vi "RT Controller.vi"() -> ()   [LabVIEW 2017]
uses:
  <vilib>/LabVIEW Targets/FPGA/cRIO/shared/nicrio_ModuleControls/nicrio_cRIO-9775_RecordDataRates4ChansRing.ctl
  <vilib>/FPGAPlugInAG/cRIO-9063/niLvFpga_Open_cRIO-9063.vi
  <vilib>/rvi/interface/common/dynamic/niFpgaDynamicAddResources.vi
  <vilib>/FPGAPlugInAG/Dynamic/niLvFpga_Reset_Dynamic.vi
  <vilib>/Utility/error.llb/Error Cluster From Error Code.vi
  <vilib>/rvi/errors/niLvFpgaAdjustHostInterfaceError.vi
  <vilib>/FPGAPlugInAG/Dynamic/niLvFpga_Run_Dynamic.vi
  <vilib>/RVI Host/nirviSupport.llb/nirviErrorClusterFromErrorCode.vi
  <vilib>/FPGAPlugInAG/Dynamic/niLvFpga_Close_Dynamic.vi
  <vilib>/rvi/interface/nirviOpenFPGA/nirviOpenFPGA.xnode
  FPGA Bitfiles/Mainproject_FPGATarget_Icreadoutclocked_gpGzf-zKHUg.lvbitx
  Ic readout_clocked_dist.vi
  <vilib>/rvi/interface/nirviMethod/nirviMethod.xnode
  <vilib>/rvi/interface/nirviReadWriteControl/nirviReadWriteControl.xnode
  <vilib>/rvi/interface/nirviCloseFPGA/nirviCloseFPGA.xnode
  <resource>/objmgr/ni.dex.rc
  <vilib>/rvi/interface/nirviMethod/StockFPGA_InlinedMethodWaitForSingleIRQ.vi
  <vilib>/FPGAPlugInAG/Dynamic/niLvFpga_WaitOnIrq_Dynamic.vi
  <vilib>/FPGAPlugInAG/Dynamic/niLvFpga_AcknowledgeIrq_Dynamic.vi
  <vilib>/FPGAPlugInAG/Dynamic/niLvFpga_ReadFifo_Dynamic.vi
  <vilib>/rvi/errors/niLvFpgaMergeErrorWithErrorCode.vi
  NiFpgaLv.dll
  <vilib>/rvi/interface/Simulation/niFpgaSimulationCallBeginRW.vi
panel:
  in  "Count ms":u32=15
  out "error out":errorcluster
  in  "Parameters":T2 {"Record Data Rate" items=["20.000 MS/s (NI 9775)"=1, "10.00 MS/s (NI 9775)"=2, "6.667 MS/s (NI 9775)"=3, "5.000 MS/s (NI 9775)"=4, "2.500 MS/s (NI 9775)"=8, "1.667 MS/s (NI 9775)"=12, "1.250 MS/s (NI 9775)"=16, "1.000 MS/s (NI 9775)"=20, "833.333 KS/s (NI 9775)"=24, "714.286 KS/s (NI 9775)"=28, "625.000 KS/s (NI 9775)"=32, "555.556 KS/s (NI 9775)"=36, "500.000 KS/s (NI 9775)"=40, "454.545 KS/s (NI 9775)"=44, "416.667 KS/s (NI 9775)"=48, "384.615 KS/s (NI 9775)"=52, "357.143 KS/s (NI 9775)"=56, "333.333 KS/s (NI 9775)"=60, "312.500 KS/s (NI 9775)"=64, "294.118 KS/s (NI 9775)"=68, "277.778 KS/s (NI 9775)"=72, "263.158 KS/s (NI 9775)"=76, "250.000 KS/s (NI 9775)"=80, "238.095 KS/s (NI 9775)"=84, "227.273 KS/s (NI 9775)"=88, "217.391 KS/s (NI 9775)"=92, "208.333 KS/s (NI 9775)"=96, "200.000 KS/s (NI 9775)"=100, "192.308 KS/s (NI 9775)"=104, "185.185 KS/s (NI 9775)"=108, "178.571 KS/s (NI 9775)"=112, "172.414 KS/s (NI 9775)"=116, "166.667 KS/s (NI 9775)"=120, "161.290 KS/s (NI 9775)"=124, "156.250 KS/s (NI 9775)"=128, "151.515 KS/s (NI 9775)"=132, "147.059 KS/s (NI 9775)"=136, "142.857 KS/s (NI 9775)"=140, "138.889 KS/s (NI 9775)"=144, "135.135 KS/s (NI 9775)"=148, "131.579 KS/s (NI 9775)"=152, "128.205 KS/s (NI 9775)"=156, "125.000 KS/s (NI 9775)"=160, "121.951 KS/s (NI 9775)"=164, "119.048 KS/s (NI 9775)"=168, "116.279 KS/s (NI 9775)"=172, "113.636 KS/s (NI 9775)"=176, "111.111 KS/s (NI 9775)"=180, "108.696 KS/s (NI 9775)"=184, "106.383 KS/s (NI 9775)"=188, "104.167 KS/s (NI 9775)"=192, "102.041 KS/s (NI 9775)"=196, "100.000 KS/s (NI 9775)"=200, "50.000 KS/s (NI 9775)"=400, "33.333 KS/s (NI 9775)"=600, "25.000 KS/s (NI 9775)"=800, "20.000 KS/s (NI 9775)"=1000, "16.667 KS/s (NI 9775)"=1200, "14.286 KS/s (NI 9775)"=1400, "12.500 KS/s (NI 9775)"=1600, "11.111 KS/s (NI 9775)"=1800, "10.000 KS/s (NI 9775)"=2000, "9.091 KS/s (NI 9775)"=2200, "8.333 KS/s (NI 9775)"=2400, "7.692 KS/s (NI 9775)"=2600, "7.143 KS/s (NI 9775)"=2800, "6.667 KS/s (NI 9775)"=3000, "6.250 KS/s (NI 9775)"=3200, "5.882 KS/s (NI 9775)"=3400, "5.556 KS/s (NI 9775)"=3600, "5.000 KS/s (NI 9775)"=4000, "4.762 KS/s (NI 9775)"=4200, "4.545 KS/s (NI 9775)"=4400, "4.348 KS/s (NI 9775)"=4600, "4.167 KS/s (NI 9775)"=4800, "4.000 KS/s (NI 9775)"=5000, "3.846 KS/s (NI 9775)"=5200, "3.571 KS/s (NI 9775)"=5600, "3.333 KS/s (NI 9775)"=6000, "3.125 KS/s (NI 9775)"=6400, "2.941 KS/s (NI 9775)"=6800, "2.778 KS/s (NI 9775)"=7200, "2.632 KS/s (NI 9775)"=7600, "2.500 KS/s (NI 9775)"=8000, "2.381 KS/s (NI 9775)"=8400, "2.273 KS/s (NI 9775)"=8800, "2.174 KS/s (NI 9775)"=9200, "2.083 KS/s (NI 9775)"=9600, "2.000 KS/s (NI 9775)"=10000, "1.923 KS/s (NI 9775)"=10400, "1.852 KS/s (NI 9775)"=10800, "1.786 KS/s (NI 9775)"=11200, "1.724 KS/s (NI 9775)"=11600, "1.667 KS/s (NI 9775)"=12000, "1.613 KS/s (NI 9775)"=12400, "1.563 KS/s (NI 9775)"=12800, "1.515 KS/s (NI 9775)"=13200, "1.471 KS/s (NI 9775)"=13600, "1.429 KS/s (NI 9775)"=14000, "1.389 KS/s (NI 9775)"=14400, "1.351 KS/s (NI 9775)"=14800, "1.316 KS/s (NI 9775)"=15200, "1.282 KS/s (NI 9775)"=15600, "1.250 KS/s (NI 9775)"=16000, "1.220 KS/s (NI 9775)"=16400, "1.190 KS/s (NI 9775)"=16800, "1.163 KS/s (NI 9775)"=17200, "1.136 KS/s (NI 9775)"=17600, "1.111 KS/s (NI 9775)"=18000, "1.087 KS/s (NI 9775)"=18400, "1.064 KS/s (NI 9775)"=18800, "1.042 KS/s (NI 9775)"=19200, "1.020 KS/s (NI 9775)"=19600, "1.000 KS/s (NI 9775)"=20000, "0.980 KS/s (NI 9775)"=20400, "0.962 KS/s (NI 9775)"=20800, "0.943 KS/s (NI 9775)"=21200, "0.926 KS/s (NI 9775)"=21600, "0.909 KS/s (NI 9775)"=22000, "0.893 KS/s (NI 9775)"=22400, "0.877 KS/s (NI 9775)"=22800, "0.862 KS/s (NI 9775)"=23200, "0.847 KS/s (NI 9775)"=23600, "0.833 KS/s (NI 9775)"=24000, "0.820 KS/s (NI 9775)"=24400, "0.806 KS/s (NI 9775)"=24800, "0.794 KS/s (NI 9775)"=25200, "0.781 KS/s (NI 9775)"=25600, "0.694 KS/s (NI 9775)"=28800, "0.625 KS/s (NI 9775)"=32000, "0.568 KS/s (NI 9775)"=35200, "0.521 KS/s (NI 9775)"=38400, "0.446 KS/s (NI 9775)"=44800, "0.391 KS/s (NI 9775)"=51200, "0.347 KS/s (NI 9775)"=57600, "0.313 KS/s (NI 9775)"=64000]}
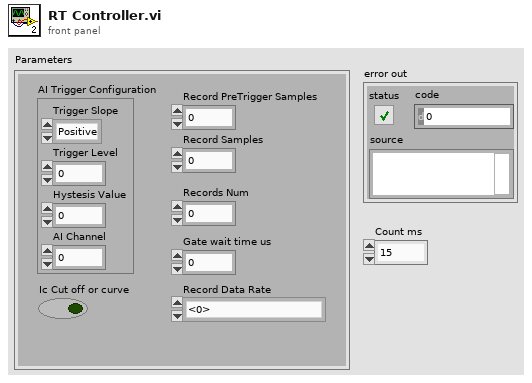
[diagram p1: front panel]
types:
  T1 = typedef "nicrio_cRIO-9775_RecordDataRates4ChansRing.ctl" = u16
  T2 = cluster{"Records Num":i32, "AI Trigger Configuration":cluster{"Trigger Slope":enum8{"Positive", "Negative"}, "Trigger Level":fxp<+/-,17,5>, "Hystesis Value":fxp<+,16,4>, "AI Channel":u8}, "Record PreTrigger Samples":u32, "Record Samples":u32, "Ic Cut off or curve":bool, "Gate wait time us":u32, "Record Data Rate":T1}
  T3 = cluster{"Trigger Slope":enum8{"Positive", "Negative"}, "Trigger Level":fxp<+/-,17,5>, "Hystesis Value":fxp<+,16,4>, "AI Channel":u8}
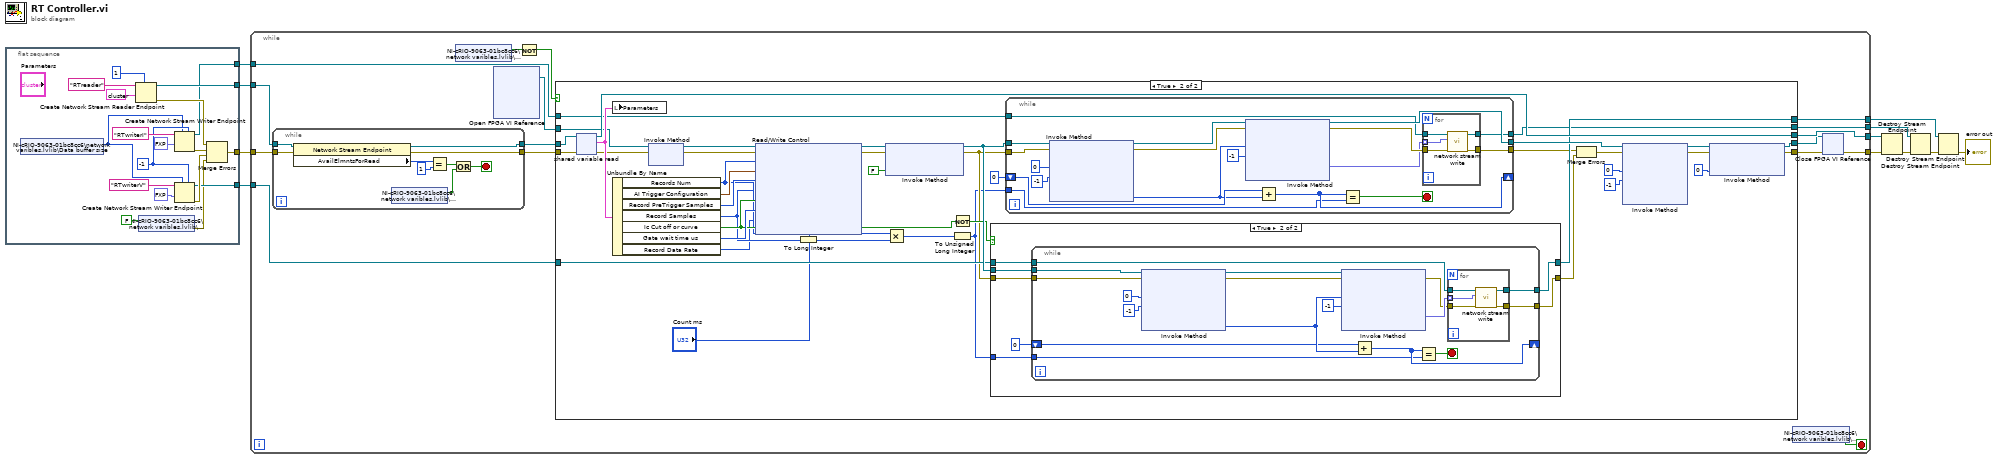
[diagram p0: block diagram]
diagram:
  n1 = flat-sequence {
    tunnel: [w27] -> w11
    tunnel: [w17] -> w10
    tunnel: [w16] -> w5
    tunnel: [w15] -> w4
    frame #0 {
      w22 = -1 ("timeout in ms (-1)")
      n2 = shared-variable "NI-cRIO-9063-01bc8cc6\\network varibles.lvlib\\Data buffer size"() -> (w21:i32)  [unwired: 1 in, 1 out]
      n3 = Create Network Stream Reader Endpoint(7:1 ("reader buffer size"), 9:T2 {"Records Num"=0, "AI Trigger Configuration"={"Trigger Slope"=enum."Positive", "Trigger Level"=0.0, "Hystesis Value"=0.0, "AI Channel"=0}, "Record PreTrigger Samples"=0, "Record Samples"=0, "Ic Cut off or curve"=FALSE, "Gate wait time us"=0, "Record Data Rate"=1} ("Parameters 2"), 11:"RTreader" ("reader name")) -> (0:w20:errorcluster, 3:w27:refnum<k21>)  [unwired: 4 in]
      n4 = shared-variable "NI-cRIO-9063-01bc8cc6\\network varibles.lvlib\\RT Stop"(FALSE ("RT Stop")) -> (error out=w13:errorcluster)  [unwired: 1 in]
      n5 = Create Network Stream Writer Endpoint(5:w22, 7:w21, 9:fxp<+/-,17,5> 0.0, 11:"RTwriterI" ("writer name")) -> (0:w19:errorcluster, 3:w16:refnum<k21>)  [unwired: 3 in]
      n6 = Create Network Stream Writer Endpoint(5:w22, 7:w21, 9:fxp<+/-,17,5> 0.0, 11:"RTwriterV" ("writer name")) -> (0:w18:errorcluster, 3:w15:refnum<k21>)  [unwired: 3 in]
      n7 = Merge Errors(w20, w19, w18, w13) -> (w17:errorcluster)
    }
  }
  n8 = while {
    tunnel: w11 -> [w45]
    tunnel: w10 -> [w44]
    tunnel: [w30] -> w1
    tunnel: [w41] -> w9
    tunnel: w5 -> [w36]
    tunnel: w4 -> [w35]
    tunnel: [w34] -> w3
    tunnel: [w33] -> w2
    stop <- w40 stop-if-true
    n9 = while {
      tunnel: w45 -> [w154]
      tunnel: w44 -> [w153]
      tunnel: [w152] -> w43
      tunnel: [w151] -> w42
      stop <- w146 stop-if-true
      n10 = property class="Network Stream Endpoint"(reference=w154, error in=w153) -> (reference out=w152:refnum<k21>, error out=w151:errorcluster, "AvailElmntsForRead"=w150:i32)
      n11 = shared-variable "NI-cRIO-9063-01bc8cc6\\network varibles.lvlib\\RT Stop"() -> (w147:bool)  [unwired: 1 in, 1 out]
      n12 = Equal?(x=w150, y=1) -> (x = y?=w148:bool)
      n13 = Or(x=w148, y=w147) -> (x .or. y?=w146:bool)
    }
    n14 = shared-variable "NI-cRIO-9063-01bc8cc6\\network varibles.lvlib\\RT Stop"() -> (w39:bool)  [unwired: 1 in, 1 out]
    n15 = xnode "Open FPGA VI Reference"() -> ("FPGA VI Reference Out"=w37:refnum<k20>)  [unwired: 2 in, 1 out]
    n16 = Not(x=w39) -> (.not. x?=w38:bool)
    n17 = case shown="True" w38 {
      tunnel: w43 -> [w49 w86]
      tunnel: w42 -> [w50 w85]
      tunnel: [w48 w76] -> w32
      tunnel: [w50 w75] -> w31
      tunnel: [w49 w74] -> w41
      tunnel: w37 -> [w48 w67]
      tunnel: w36 -> [w47 w59]
      tunnel: w35 -> [w46 w61]
      tunnel: [w47 w58] -> w34
      tunnel: [w46 w60] -> w33
      frame False {
      }
      frame True {
        n18 = shared-variable-read(w86, w85) -> (w74:refnum<k21>, w66:errorcluster, w84:T2)  [unwired: 1 in, 1 out]
        n19 = local write "Parameters"(w84) -> ()
        n20 = Unbundle By Name(w84) -> ("Records Num"=w65:i32, "AI Trigger Configuration"=w88:T3, "Record PreTrigger Samples"=w87:u32, "Record Samples"=w64:u32, "Ic Cut off or curve"=w70:bool, "Gate wait time us"=w83:u32, "Record Data Rate"=w56:T1)
        n21 = xnode "Invoke Method"("FPGA VI Reference In"=w67, "error in"=w66) -> ("FPGA VI Reference Out"=w90:refnum<k20>, "error out"=w68:errorcluster)
        n22 = xnode "Read/Write Control"("FPGA VI Reference In"=w90, "error in"=w68, "Records Num"=w65, "AI Trigger Configuration"=w88, "Record PreTrigger Samples"=w87, "Record Samples"=w64, "Ic Cut off or curve"=w70, "Gate wait time us"=w83, "Record Data Rate"=w56, "Count ms"="Count ms") -> ("FPGA VI Reference Out"=w91:refnum<k20>, "error out"=w52:errorcluster)
        n23 = To Long Integer(number=w64) -> (32bit integer=w63:i32)
        n24 = xnode "Invoke Method"("FPGA VI Reference In"=w91, "error in"=w52, "Wait Until Done (F)"=FALSE) -> ("FPGA VI Reference Out"=w73:refnum<k20>, "error out"=w54:errorcluster)
        n25 = Multiply(x=w65, y=w63) -> (x*y=w62:i32)
        n26 = Not(x=w70) -> (.not. x?=w69:bool)
        n27 = To Unsigned Long Integer(number=w62) -> (unsigned 32bit integer=w53:u32)
        n28 = case shown="True" w69 {
          tunnel: w73 -> [_ w123]
          tunnel: [w115 w117] -> w72
          tunnel: w61 -> [w116 w122]
          tunnel: [w116 w118] -> w60
          tunnel: w54 -> [w115 w120]
          tunnel: w53 -> [_ w119]
          frame False {
          }
          frame True {
            n29 = while {
              tunnel: w123 -> [w131]
              tunnel: w122 -> [w130]
              shift-right: [w127] -> _
              shift-left: u32 0 ("Number of Elements") -> [w129]
              tunnel: w120 -> [w128]
              tunnel: w119 -> [w126]
              tunnel: [w125] -> w118
              tunnel: [w124] -> w117
              stop <- w132 stop-if-true
              n30 = xnode "Invoke Method"("FPGA VI Reference In"=w131, "error in"=w128, "Number of Elements"=u32 0, "Timeout (ms)"=-1) -> ("FPGA VI Reference Out"=w138:refnum<k20>, "error out"=w139:errorcluster, "Elements Remaining"=w140:u32)  [unwired: 1 out]
              n31 = xnode "Invoke Method"("FPGA VI Reference In"=w138, "error in"=w139, "Number of Elements"=w140, "Timeout (ms)"=-1) -> ("error out"=w136:errorcluster, "Data"=w137:fxp<+/-,17,5>[])  [unwired: 2 out]
              n32 = Add(x=w129, y=w140) -> (x+y=w127:u32)
              n33 = Equal?(x=w127, y=w126) -> (x = y?=w132:bool)
              n34 = for {
                tunnel: w136 -> [w145]
                tunnel: w137 -> [w144] mode=indexing
                tunnel: [w143] -> w125
                tunnel: [w142] -> w124
                tunnel: w130 -> [w141]
                n35 = call "network stream write.vi"("error in (no error)"=w145, "Data"=w144, "endpoint in"=w141) -> ("error out"=w142:errorcluster, "endpoint out"=w143:refnum<k21>)  [unwired: 7 in]
              }
            }
          }
        }
        n36 = while {
          tunnel: w59 -> [w107]
          tunnel: [w104] -> w58
          tunnel: w73 -> [w102]
          tunnel: [w108] -> w82
          tunnel: w54 -> [w100]
          tunnel: [w103] -> w57
          shift-right: [w94] -> _
          shift-left: u32 0 ("Number of Elements") -> [w96]
          tunnel: w53 -> [w93]
          stop <- w92 stop-if-true
          n37 = xnode "Invoke Method"("FPGA VI Reference In"=w102, "error in"=w100, "Number of Elements"=u32 0, "Timeout (ms)"=-1) -> ("FPGA VI Reference Out"=w101:refnum<k20>, "error out"=w99:errorcluster, "Elements Remaining"=w95:u32)  [unwired: 1 out]
          n38 = xnode "Invoke Method"("FPGA VI Reference In"=w101, "error in"=w99, "Number of Elements"=w95, "Timeout (ms)"=-1) -> ("FPGA VI Reference Out"=w108:refnum<k20>, "error out"=w106:errorcluster, "Data"=w105:fxp<+/-,17,5>[])  [unwired: 1 out]
          n39 = Add(x=w96, y=w95) -> (x+y=w94:u32)
          n40 = Equal?(x=w94, y=w93) -> (x = y?=w92:bool)
          n41 = for {
            tunnel: w107 -> [w114]
            tunnel: w106 -> [w113]
            tunnel: w105 -> [w112] mode=indexing
            tunnel: [w111] -> w104
            tunnel: [w110] -> w103
            n42 = call "network stream write.vi"("error in (no error)"=w113, "Data"=w112, "endpoint in"=w114) -> ("error out"=w110:errorcluster, "endpoint out"=w111:refnum<k21>)  [unwired: 7 in]
          }
        }
        n43 = Merge Errors(w57, w72) -> (w71:errorcluster)
        n44 = xnode "Invoke Method"("FPGA VI Reference In"=w82, "error in"=w71, "IRQ Number(s)"=0, "Timeout (ms)"=-1) -> ("FPGA VI Reference Out"=w79:refnum<k20>, "error out"=w78:errorcluster)  [unwired: 2 out]
        n45 = xnode "Invoke Method"("FPGA VI Reference In"=w79, "error in"=w78, "IRQ Number(s)"=0) -> ("FPGA VI Reference Out"=w76:refnum<k20>, "error out"=w75:errorcluster)
      }
    }
    n46 = shared-variable "NI-cRIO-9063-01bc8cc6\\network varibles.lvlib\\RT Stop"() -> (w40:bool)  [unwired: 1 in, 1 out]
    n47 = xnode "Close FPGA VI Reference"("FPGA VI Reference In"=w32, "error in"=w31) -> ("error out"=w30:errorcluster)
  }
  n48 = Destroy Stream Endpoint(8:w1, 11:w9) -> (0:w8:errorcluster)
  n49 = Destroy Stream Endpoint(8:w8, 11:w3) -> (0:w7:errorcluster)
  n50 = Destroy Stream Endpoint(8:w7, 11:w2) -> (0:→"error out":errorcluster)
